vi "Quit Application.vi"(8 "error in (no error)":errorcluster, 10 "window name (\"\")":string, 11 "window refnum (NaWR)":T1) -> (0 "error out":errorcluster)   [LabVIEW 2020, in "MacroAssert.lvlib" / "Win Util.lvlib"]
doc: "This VI will close the application identified by window ID in or by the name of the application window. Note that the window to be closed must have no owner or parent window.\n\nFor example, this VI will not work if sent to another LabVIEW VI window - use LabVIEW's built-in Exit function to quit LabVIEW."
uses:
  Win Util.lvlib
  Window Refnum.ctl
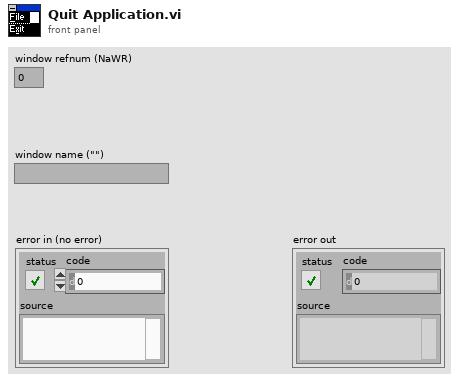
[diagram p1: front panel]
types:
  T1 = typedef "MacroAssert.lvlib/Win Util.lvlib/Window Refnum.ctl" = u64
  T2 = enum8{"Maximize Window", "Minimize Window", "Show Task List", "Start Screen Saver", "Quit Application"}
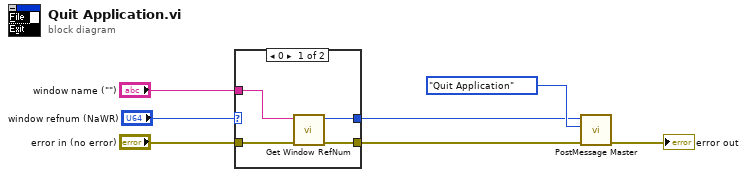
[diagram p0: block diagram]
diagram:
  n1 = case shown="0" "window refnum (NaWR)" {
    selector: "window refnum (NaWR)" -> [_ w13]
    tunnel: "error in (no error)" -> [w11 w12]
    tunnel: [w10 w13] -> w5
    tunnel: [w9 w12] -> w4
    tunnel: "window name (\"\")" -> [w8 _]
    frame 0 {
      n2 = call "Get Window RefNum.vi"("error in"=w11, "window name (\"\")"=w8) -> ("error out"=w9:errorcluster, "window refnum (NaWR)"=w10:T1)  [unwired: 6 in]
    }
    frame Default {
    }
  }
  n3 = call "PostMessage Master.vi"("error in"=w4, "Function"=T2."Quit Application", "window refnum"=w5) -> ("error out"=→"error out":errorcluster)  [unwired: 7 in, 1 out]
